vi "Test_Image_construct.vi"() -> ()   [LabVIEW 2015]
panel:
  out "Image Array Out":dbl[][](array[numeric]) format="%.2f"
  in  "Acq.Point":u16[](array[numeric])
  in  "Image Array":dbl[][](array[numeric])
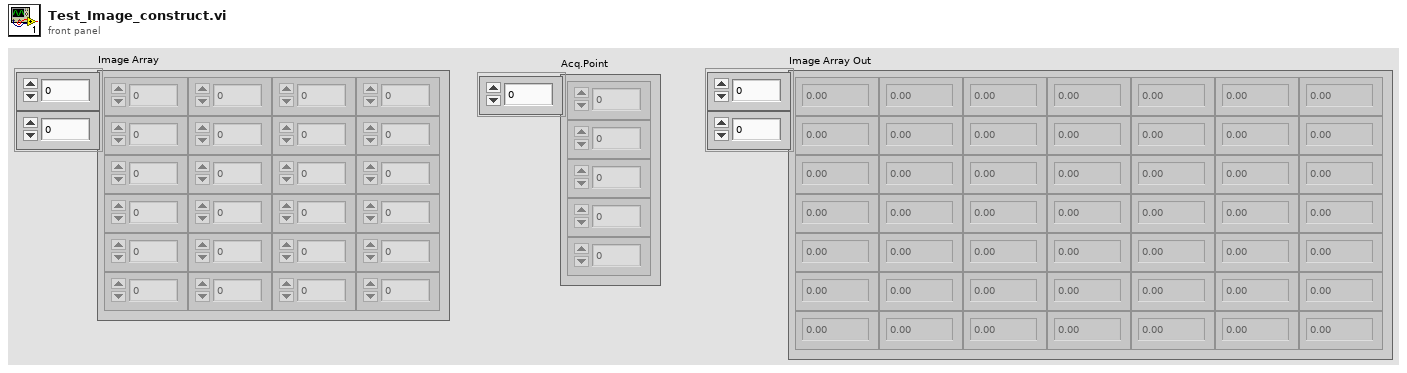
[diagram p1: front panel]
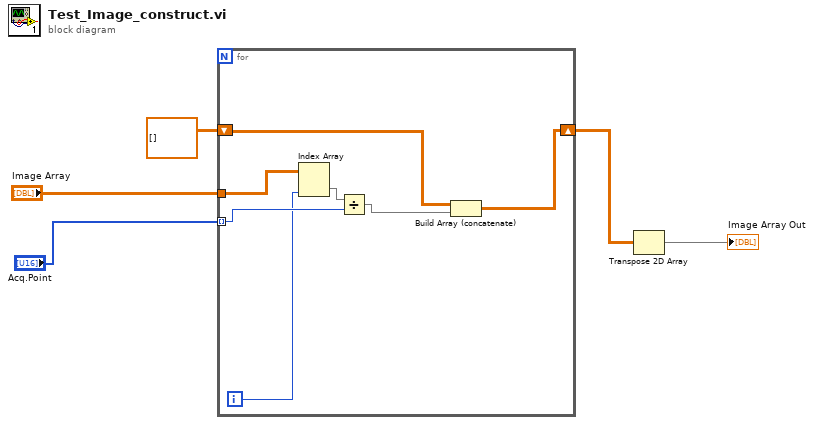
[diagram p0: block diagram]
diagram:
  n1 = for {
    tunnel: "Image Array" -> [w11]
    tunnel: "Acq.Point" -> [w12] mode=indexing
    shift-right: [w6] -> w2
    shift-left: dbl[][] [] -> [w8]
    i -> [w10]
    n2 = Index Array(array=w11, index (col)=w10) -> (element=w9:dbl[])  [unwired: 1 in]
    n3 = Divide(x=w9, y=w12) -> (x/y=w7:dbl[])
    n4 = Build Array (concatenate)(w8, w7) -> (w6:dbl[][])
  }
  n5 = Transpose 2D Array(2D array=w2) -> (transposed array=→"Image Array Out":dbl[][])
